vi "CMI ADS127L21 - Start Sampling.vi"(8 "error in (no error)":errorcluster, 11 "session in":T1 {"channels"."Channel" min=1 max=8 step=1}) -> (0 "error out":errorcluster, 3 "session out":T1 {"channels"."Channel" min=1 max=8 step=1})   [LabVIEW 2020]
doc: "Start ADC sampling with current configuration. Must be done before recording and after any configuration change."
uses:
  CMI ADS127L21 - Session.ctl
  CMI ADS127L21 - Record Channel.ctl
  CMI ADS127L21 - Input Range.ctl
  CMI ADS127L21 - Input Mode.ctl
  CMI ADS127L21 - Input Impedance.ctl
  CMI ADS127L21 - EXTOUT Mode.ctl
  CMI ADS127L21 - EXTOUT Polarity.ctl
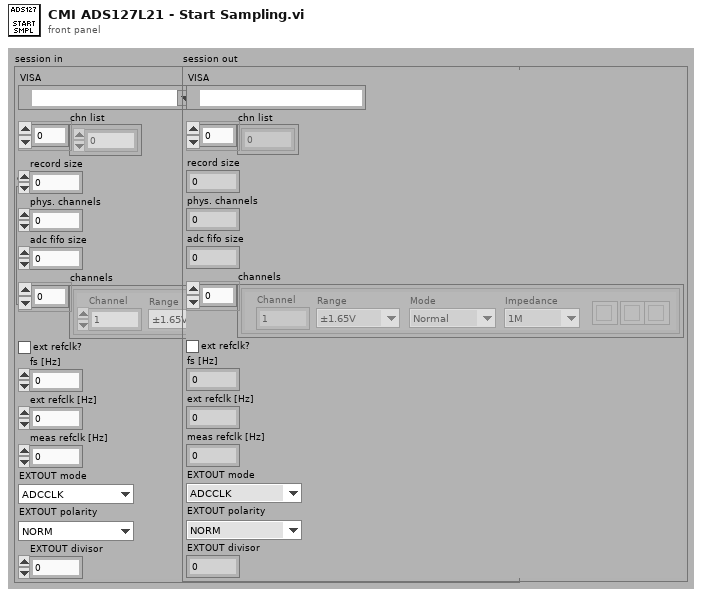
[diagram p1: front panel]
types:
  T1 = typedef "CMI ADS127L21 - Session.ctl" = cluster{"VISA":refnum<visa-resource-name>, "chn list":i32[], "record size":i32, "phys. channels":i32, "adc fifo size":i32, "channels":T2[], "ext refclk?":bool, "fs [Hz]":dbl, "ext refclk [Hz]":dbl, "meas refclk [Hz]":dbl, "EXTOUT mode":T6, "EXTOUT polarity":T7, "EXTOUT divisor":i32}
  T2 = typedef "CMI ADS127L21 - Record Channel.ctl" = cluster{"Range":T3, "Channel":i32, "Mode":T4, "Impedance":T5, "btn clr":bool, "btn up":bool, "btn down":bool}
  T3 = typedef "CMI ADS127L21 - Input Range.ctl" = enum16{"±1.65V", "±2V"}
  T4 = typedef "CMI ADS127L21 - Input Mode.ctl" = enum16{"Normal", "Inverted", "GND"}
  T5 = typedef "CMI ADS127L21 - Input Impedance.ctl" = enum16{"1M", "1k5"}
  T6 = typedef "CMI ADS127L21 - EXTOUT Mode.ctl" = enum16{"ADCCLK", "REFCLK", "SMPLCLK", "FIRST"}
  T7 = typedef "CMI ADS127L21 - EXTOUT Polarity.ctl" = enum16{"NORM", "INV"}
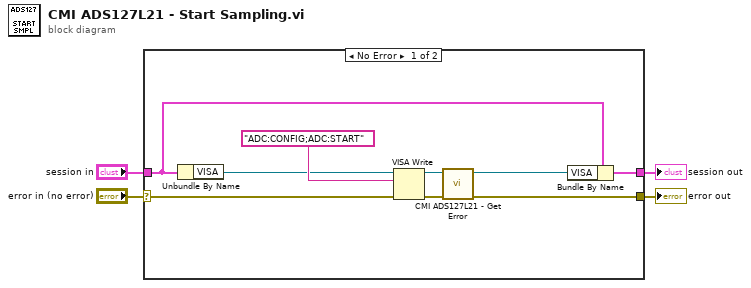
[diagram p0: block diagram]
diagram:
  n1 = case shown="No Error" "error in (no error)" {
    selector: "error in (no error)" -> [w9 w15]
    tunnel: "session in" -> [w5 w14]
    tunnel: [w6 w14] -> w3
    tunnel: [w10 w15] -> w2
    frame No Error {
      n2 = Unbundle By Name(w5) -> ("VISA"=w7:refnum<visa-resource-name>)
      n3 = VISA Write(VISA resource name=w7, write buffer="ADC:CONFIG;ADC:START" ("format string"), error in (no error)=w9) -> (VISA resource name out=w12:refnum<visa-resource-name>, error out=w13:errorcluster)  [unwired: 1 out]
      n4 = call "CMI ADS127L21 - Get Error.vi"("error in (no error)"=w13, "VISA in"=w12) -> ("error out"=w10:errorcluster, "VISA out"=w11:refnum<visa-resource-name>)  [unwired: 8 in]
      n5 = Bundle By Name(cluster=w5, "VISA"=w11) -> (w6:T1)
    }
    frame Error {
    }
  }
  "error out" <- w2
  "session out" <- w3
